vi "open.vi"(8 "error in (no error)":errorcluster) -> (0 "error out":errorcluster, 2 "Device":string, 3 "VISA resource name out":refnum<visa-resource-name>)   [LabVIEW 2009]
uses:
  <vilib>/Instr/_visa.llb/VISA Configure Serial Port (Instr).vi
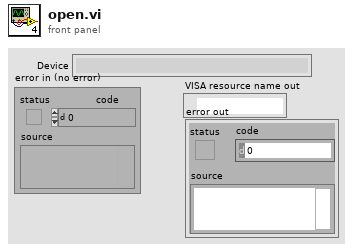
[diagram p1: front panel]
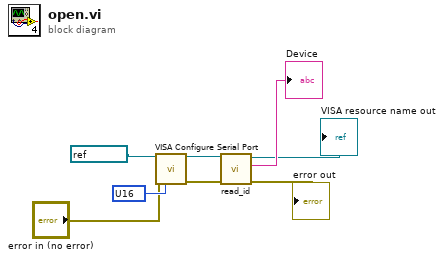
[diagram p0: block diagram]
diagram:
  w7 = u16 ? items=["1.0", "1.5", "2.0"] ("stop bits (10: 1 bit)")
  n1 = call-poly "VISA Configure Serial Port"("VISA resource name"=refnum<visa-resource-name> ?, "error in (no error)"="error in (no error)", "stop bits (10: 1 bit)"=w7) -> ("VISA resource name out"=w6:refnum<visa-resource-name>, "error out"=w5:errorcluster)  [unwired: 11 in]
  n2 = call "read_id.vi"("error in (no error)"=w5, "VISA resource name in"=w6) -> ("error out"=→"error out":errorcluster, "ID string"=→"Device":string, "VISA resource name out"=→"VISA resource name out":refnum<visa-resource-name>)  [unwired: 7 in]
